vi "create data file.vi"(5 "Time":string, 6 "end string":string, 7 "Ext name":string=".dat", 8 "error in (no error)":errorcluster, 9 "Sample Name":string, 10 "Measurement Name":string="-DAQ_IV-", 11 "base path":path) -> (0 "error out":errorcluster, 3 "appended path":path, 4 "file name":string)   [LabVIEW 2024]
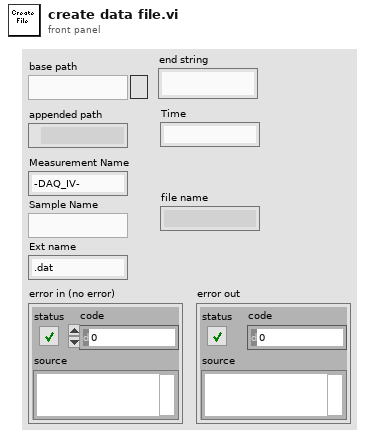
[diagram p1: front panel]
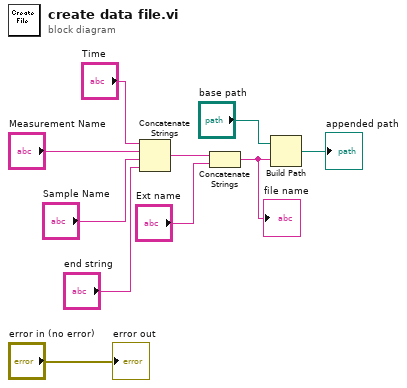
[diagram p0: block diagram]
diagram:
  n1 = Concatenate Strings("Time", "Measurement Name", "Sample Name", "end string") -> (w7:string)
  n2 = Concatenate Strings(w7, "Ext name") -> (w8:string)
  "file name" <- w8
  n3 = Build Path(base path="base path", name or relative path=w8) -> (appended path=→"appended path":path)
  "error out" <- "error in (no error)"
